vi "Set-properties.vi"(5 "Sender type":string, 7 "Sender ID":i32, 8 "error in (no error)":errorcluster, 9 "Send time":dbl, 10 "Receivers":string[](array[string]), 11 "Message in":refnum<class "Message.lvclass">) -> (0 "error out":errorcluster, 3 "Message out":refnum<class "Message.lvclass">)   [LabVIEW 2013, in "Messages.lvlib" / "Message.lvclass"]
uses:
  Message.lvclass
  Message.lvclass/Message.ctl
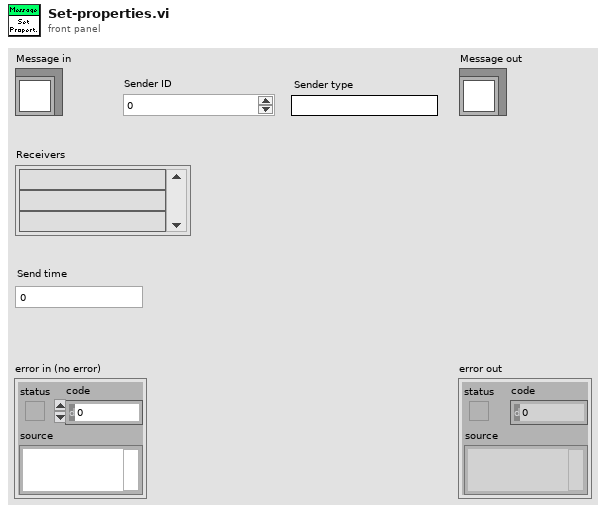
[diagram p1: front panel]
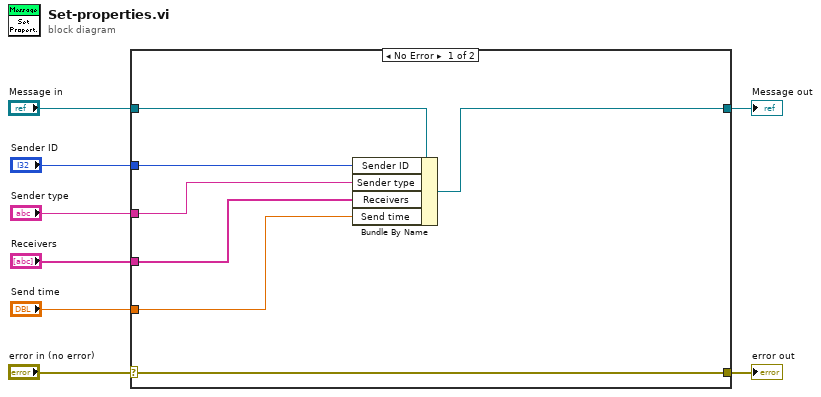
[diagram p0: block diagram]
diagram:
  n1 = case shown="No Error" "error in (no error)" {
    selector: "error in (no error)" -> [w15 w17]
    tunnel: [w15 w17] -> w7
    tunnel: [w9 w16] -> w5
    tunnel: "Message in" -> [w10 w16]
    tunnel: "Sender ID" -> [w14 _]
    tunnel: "Sender type" -> [w13 _]
    tunnel: "Receivers" -> [w12 _]
    tunnel: "Send time" -> [w11 _]
    frame No Error {
      n2 = Bundle By Name(cluster=w10, "Sender ID"=w14, "Sender type"=w13, "Receivers"=w12, "Send time"=w11) -> (w9:refnum<class "Message.lvclass">)
    }
    frame Error {
    }
  }
  "error out" <- w7
  "Message out" <- w5
